vi "Write Allele-Bit.vi"(8 "error in (no error)":errorcluster, 10 "Allele-Bit":T1, 11 "Binary Gene in":refnum<class "Binary Gene.lvclass">) -> (0 "error out":errorcluster, 3 "Binary Gene out":refnum<class "Binary Gene.lvclass">)   [LabVIEW 2016, in "Binary Gene.lvclass"]
uses:
  Binary Gene.lvclass
  _typedefs/BinaryGene_Allele.ctl
  Binary Gene.lvclass/Binary Gene.ctl
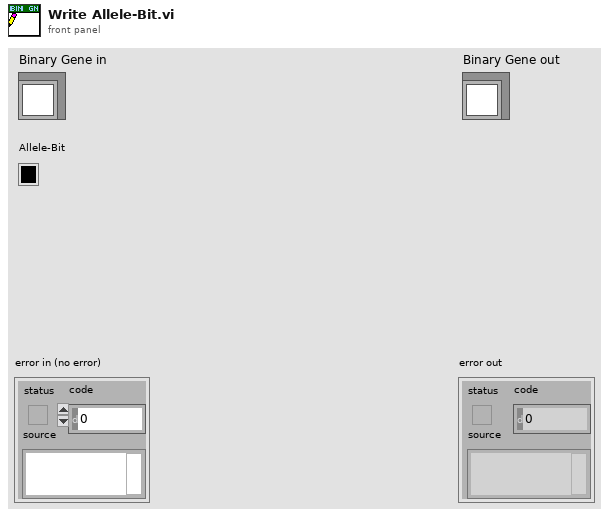
[diagram p1: front panel]
types:
  T1 = typedef "Binary Gene.lvclass/BinaryGene_Allele.ctl" = bool
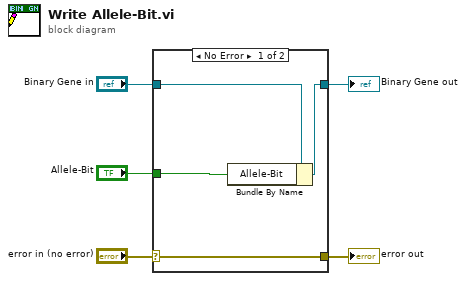
[diagram p0: block diagram]
diagram:
  n1 = case shown="No Error" "error in (no error)" {
    selector: "error in (no error)" -> [w9 w10]
    tunnel: [w9 w10] -> w4
    tunnel: [w7 w11] -> w2
    tunnel: "Binary Gene in" -> [w8 w11]
    tunnel: "Allele-Bit" -> [w6 _]
    frame No Error {
      n2 = Bundle By Name(cluster=w8, "Allele-Bit"=w6) -> (w7:refnum<class "Binary Gene.lvclass">)
    }
    frame Error {
    }
  }
  "error out" <- w4
  "Binary Gene out" <- w2
